vi "test2.vi"() -> ()   [LabVIEW 2022 SP3]
panel:
  out "Change":dbl
  in  "Return change":bool
  in  "Coke":bool
  out "Product Delivered":bool
  in  "Ramen":bool
  in  "Hershey's":bool
  in  "Arizona":bool
  in  "stop":bool
  out "Credit":dbl
  in  "Dime":bool
  in  "Quarter":bool
  in  "Nickle":bool
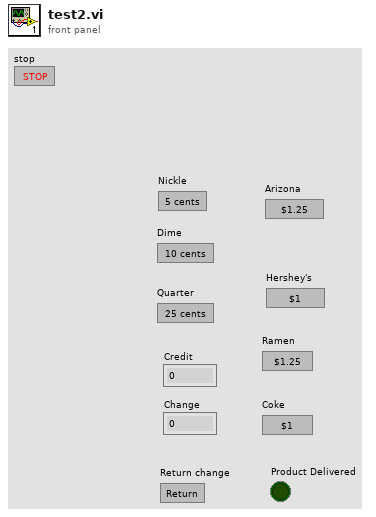
[diagram p1: front panel]
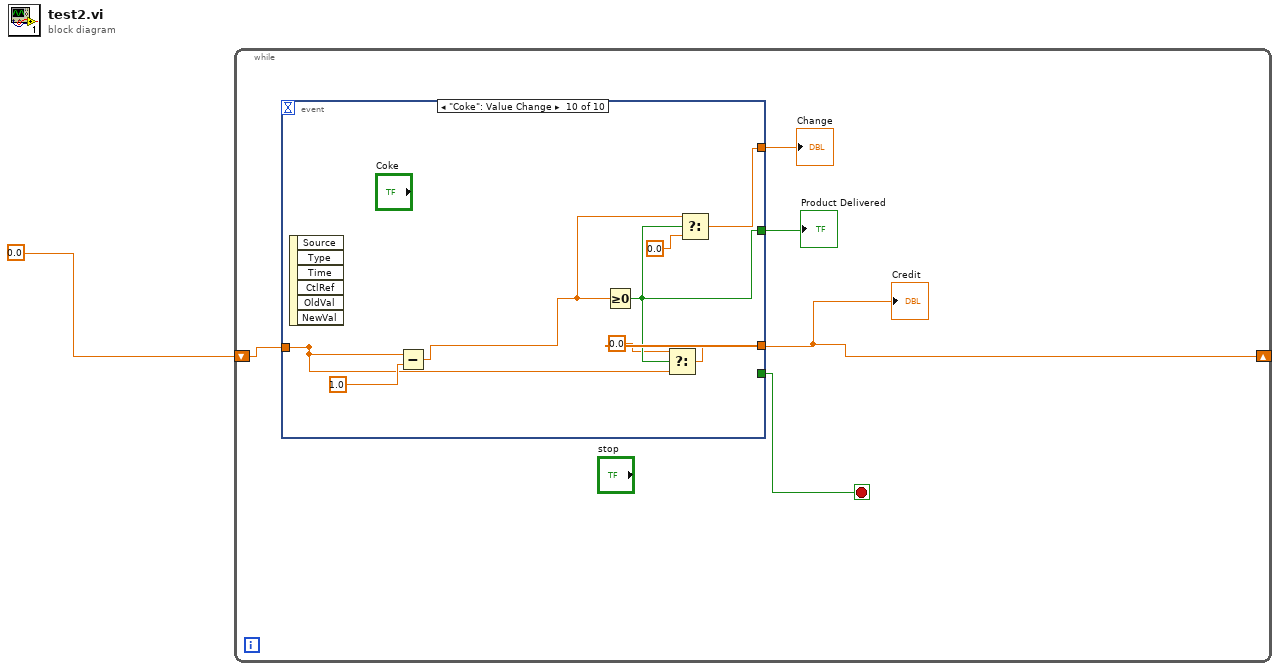
[diagram p0: block diagram]
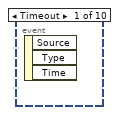
[diagram p2: hidden frame]
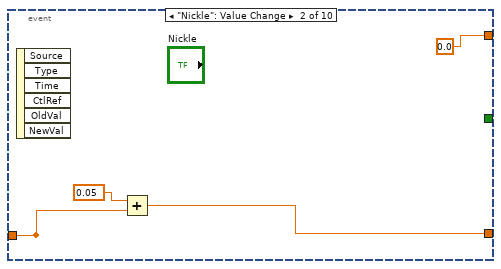
[diagram p3: hidden frame]
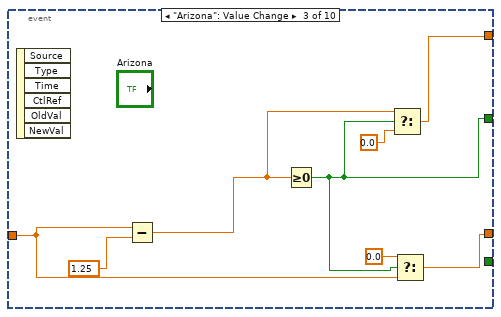
[diagram p4: hidden frame]
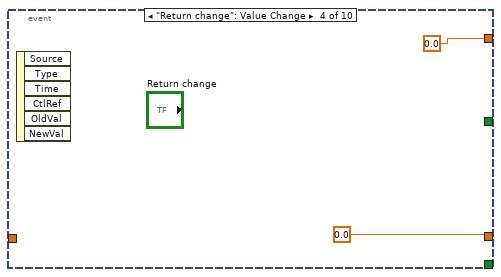
[diagram p5: hidden frame]
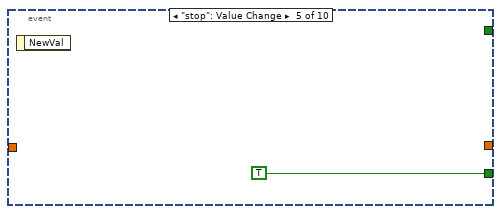
[diagram p6: hidden frame]
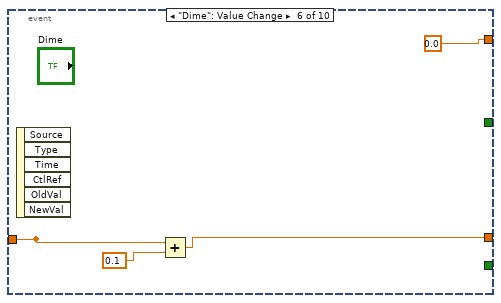
[diagram p7: hidden frame]
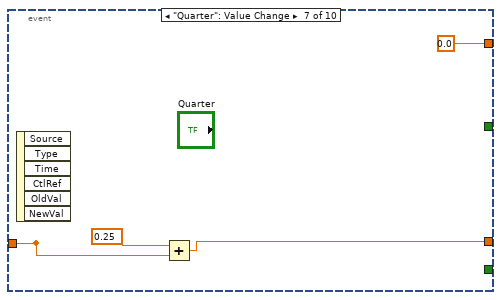
[diagram p8: hidden frame]
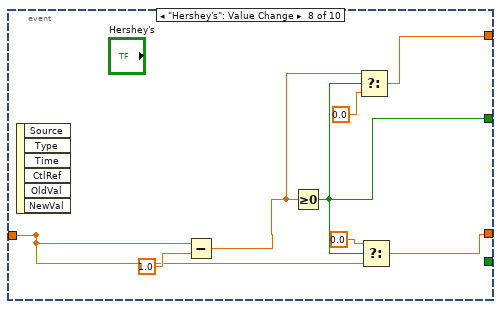
[diagram p9: hidden frame]
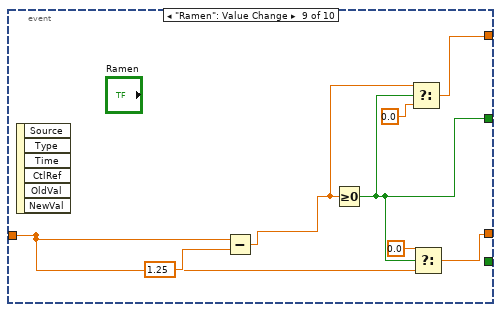
[diagram p10: hidden frame]
diagram:
  n1 = while {
    shift-right: [w5] -> _
    shift-left: 0.0 -> [w6]
    stop <- w2 stop-if-true
    n2 = event shown="[9] \"Coke\": Value Change" {
      selector: _ -> [_ _ _ _ _ _ _ _ _ _]
      dyn-events: _ -> [_ _ _ _ _ _ _ _ _ _]
      timeout: _ -> [_ _ _ _ _ _ _ _ _ _]
      tunnel: [_ w8 w12 _ _ w23 w27 w31 w39 w47] -> _
      tunnel: w6 -> [_ w8 w12 _ _ w23 w27 w31 w39 w47]
      tunnel: [_ w9 w11 0.0 _ w24 w29 w30 w38 w46] -> w5
      tunnel: [_ _ _ _ TRUE _ _ _ _ _] -> w2
      tunnel: [_ _ w13 _ _ _ _ w33 w41 w49] -> w4
      tunnel: [_ 0.0 w16 0.0 _ 0.0 0.0 w34 w44 w50] -> w3
      event Timeout {
        n3 = event-data() -> ()  [unwired: 1 in, 3 out]
      }
      event "Nickle": Value Change {
        n4 = event-data() -> ()  [unwired: 1 in, 6 out]
        n5 = Add(x=0.05, y=w8) -> (x+y=w9:dbl)
      }
      event "Arizona": Value Change {
        n6 = event-data() -> ()  [unwired: 1 in, 6 out]
        n7 = Subtract(x=w12, y=1.25) -> (x-y=w17:dbl)
        n8 = Greater Or Equal To 0?(x=w17) -> (x >= 0?=w13:bool)
        n9 = Select(t=w17, s=w13, f=0.0) -> (s? t:f=w16:dbl)
        n10 = Select(t=0.0, s=w13, f=w12) -> (s? t:f=w11:dbl)
      }
      event "Return change": Value Change {
        n11 = event-data() -> ()  [unwired: 1 in, 6 out]
      }
      event "stop": Value Change {
        n12 = event-data() -> ()  [unwired: 1 in, 1 out]
      }
      event "Dime": Value Change {
        n13 = event-data() -> ()  [unwired: 1 in, 6 out]
        n14 = Add(x=w23, y=0.1) -> (x+y=w24:dbl)
      }
      event "Quarter": Value Change {
        n15 = event-data() -> ()  [unwired: 1 in, 6 out]
        n16 = Add(x=0.25, y=w27) -> (x+y=w29:dbl)
      }
      event "Hershey's": Value Change {
        n17 = event-data() -> ()  [unwired: 1 in, 6 out]
        n18 = Subtract(x=w31, y=1.0) -> (x-y=w36:dbl)
        n19 = Greater Or Equal To 0?(x=w36) -> (x >= 0?=w33:bool)
        n20 = Select(t=w36, s=w33, f=0.0) -> (s? t:f=w34:dbl)
        n21 = Select(t=0.0, s=w33, f=w31) -> (s? t:f=w30:dbl)
      }
      event "Ramen": Value Change {
        n22 = event-data() -> ()  [unwired: 1 in, 6 out]
        n23 = Subtract(x=w39, y=1.25) -> (x-y=w42:dbl)
        n24 = Greater Or Equal To 0?(x=w42) -> (x >= 0?=w41:bool)
        n25 = Select(t=w42, s=w41, f=0.0) -> (s? t:f=w44:dbl)
        n26 = Select(t=0.0, s=w41, f=w39) -> (s? t:f=w38:dbl)
      }
      event "Coke": Value Change {
        n27 = event-data() -> ()  [unwired: 1 in, 6 out]
        n28 = Subtract(x=w47, y=1.0) -> (x-y=w51:dbl)
        n29 = Greater Or Equal To 0?(x=w51) -> (x >= 0?=w49:bool)
        n30 = Select(t=0.0, s=w49, f=w47) -> (s? t:f=w46:dbl)
        n31 = Select(t=w51, s=w49, f=0.0) -> (s? t:f=w50:dbl)
      }
    }
    "Credit" <- w5
    "Product Delivered" <- w4
    "Change" <- w3
  }
